vi "scanDeviceGlobalVars.vi"() -> ()   [LabVIEW 2014]
panel:
  in  "ScanDevice":enum16{"internal DAC", "external Python"}(ring)
  out "internalDacAvailable":bool
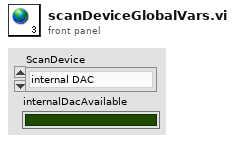
[diagram p1: front panel]
diagram:
